vi "Write Size.vi"(5 "Size":T1, 9 "String in":refnum<class "String.lvclass">) -> (3 "String out":refnum<class "String.lvclass">)   [LabVIEW 2014, in "Raspberry Pi Compatible Compiler for LabVIEW.lvlib" / "String.lvclass"]
uses:
  String.lvclass
  <vilib>/Utility/miscctls.llb/LVBoundsTypeDef.ctl
  String.lvclass/String.ctl
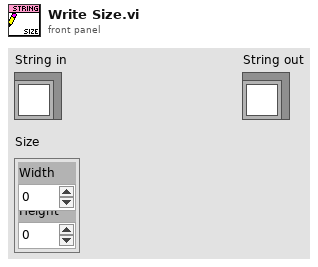
[diagram p1: front panel]
types:
  T1 = typedef "LVBoundsTypeDef.ctl" = cluster{"Width":u32, "Height":u32}
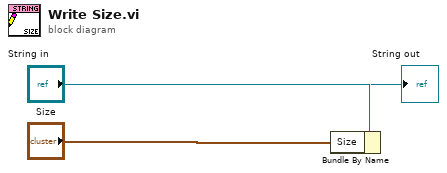
[diagram p0: block diagram]
diagram:
  n1 = Bundle By Name(cluster="String in", "Size"="Size") -> (→"String out":refnum<class "String.lvclass">)
